vi "RTM - Remove Packet Dependency.vi"(8 "error in (no error)":errorcluster, 9 "Menu hierarchy in":string[](array[string]), 11 "Node Ptr":u64 format="%.0x") -> (0 "error out":errorcluster, 1 "Menu hierarchy out":string[](array[string]), 3 "Action":T1)   [LabVIEW 2015, in "UDP-Custom-Device System Explorer.lvlib"]
uses:
  UDP-Custom-Device System Explorer.lvlib
  <vilib>/NI Veristand/Custom Device API/Custom Device RTM Dependency.ctl
  Shared/Constants.vi
  Shared/UDP-Custom-Device Shared.lvlib
  <vilib>/NI VeriStand/Custom Device API/Custom Device API.lvlib
  <vilib>/NI VeriStand/Custom Device Tools/Custom Device Utility Library/Custom Device Utility Library.lvlib
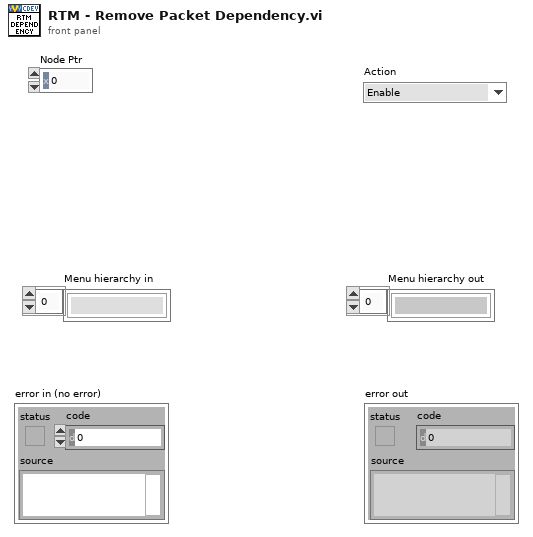
[diagram p1: front panel]
types:
  T1 = typedef "Custom Device API.lvlib/Custom Device RTM Dependency.ctl" = enum16{"Enable", "Disable", "Hide"}
  T2 = typedef "Custom Device API.lvlib/Custom Device Item Ref.ctl" = u64
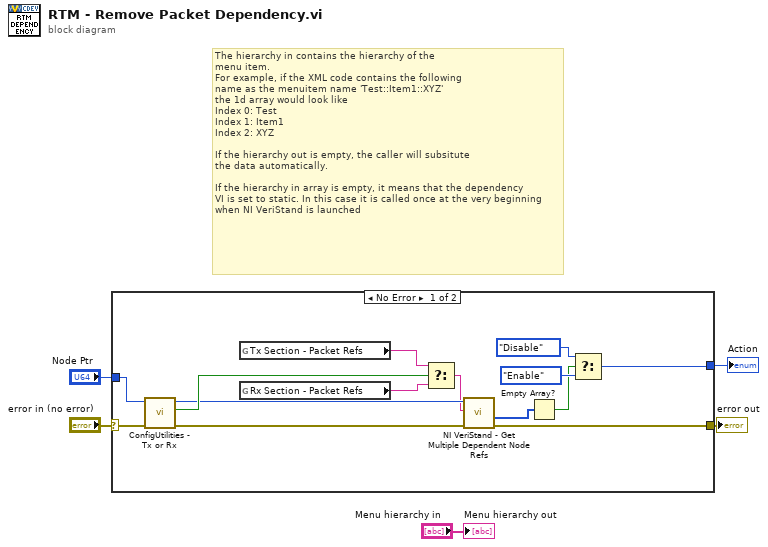
[diagram p0: block diagram]
diagram:
  # "The hierarchy in contains the hierarchy of the\nmenu item.\nFor example, if the XML code contains the following\nname as the menuitem name 'Test::Item1::XYZ'\nthe 1d array would look like\nIndex 0: Test\nIndex 1: Item1\nIndex 2: XYZ\n\nIf the hierarchy out is empty, the caller will subsitute\nthe data automatically.\n\nIf the hierarchy in array is empty, it means that the dependency\nVI is set to static. In this case it is called once at the very beginning\nwhen NI VeriStand is launched"
  n1 = case shown="No Error" "error in (no error)" {
    selector: "error in (no error)" -> [w14 w20]
    tunnel: "Node Ptr" -> [w13 _]
    tunnel: [w19 _] -> w3
    tunnel: [w11 w20] -> w1
    frame No Error {
      n2 = call "ConfigUtilities - Tx or Rx.vi"("error in (no error)"=w14, "Item Ref in"=w13) -> ("error out"=w9:errorcluster, "Tx?"=w12:bool, "Item Ref out"=w8:T2)  [unwired: 7 in]
      n3 = global read "Constants.vi" "Tx Section - Packet Refs"() -> (w16:string)
      n4 = global read "Constants.vi" "Rx Section - Packet Refs"() -> (w15:string)
      n5 = Select(t=w16, s=w12, f=w15) -> (s? t:f=w7:string)
      n6 = call <vilib>:"NI VeriStand - Get Multiple Dependent Node Refs.vi"("error in (no error)"=w9, "Base Property Name"=w7, "Item Ref in"=w8) -> ("error out"=w11:errorcluster, "Dependent Node Refs"=w10:T2[])  [unwired: 6 in, 1 out]
      n7 = Empty Array?(array=w10) -> (empty?=w6:bool)
      n8 = Select(t=Custom_Device_RTM_Dependency."Disable" ("Action"), s=w6, f=Custom_Device_RTM_Dependency."Enable" ("Action")) -> (s? t:f=w19:T1)
    }
    frame Error {
    }
  }
  "error out" <- w1
  "Action" <- w3
  "Menu hierarchy out" <- "Menu hierarchy in"
